vi "DrawGridOnMap.vi"(11 "Mission MapIn":picture) -> (3 "Mission MapOut":picture)   [LabVIEW 2014]
panel:
  out "decimal integer string":string
  out "Index":i32
  # "This Vi draws a grid on map with squares of N resolution"
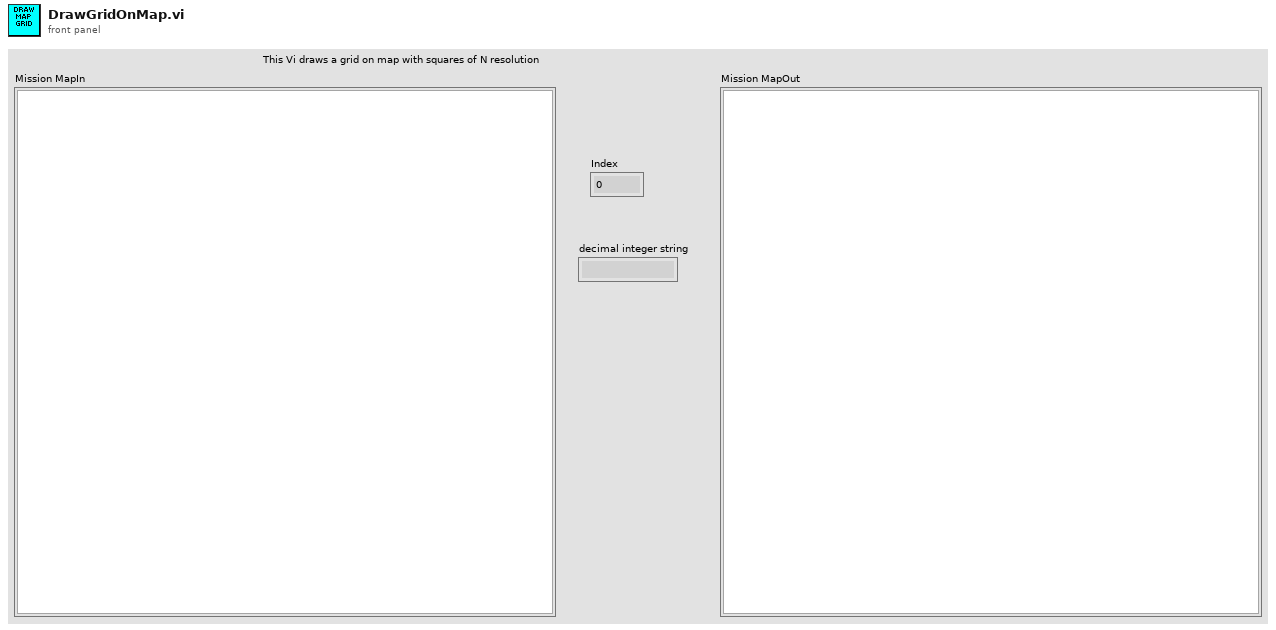
[diagram p1: front panel]
types:
  T1 = cluster{"Width":u16, "Style":enum32{"Solid", "Dash", "Dot", "DashDot", "DashDotDot"}}
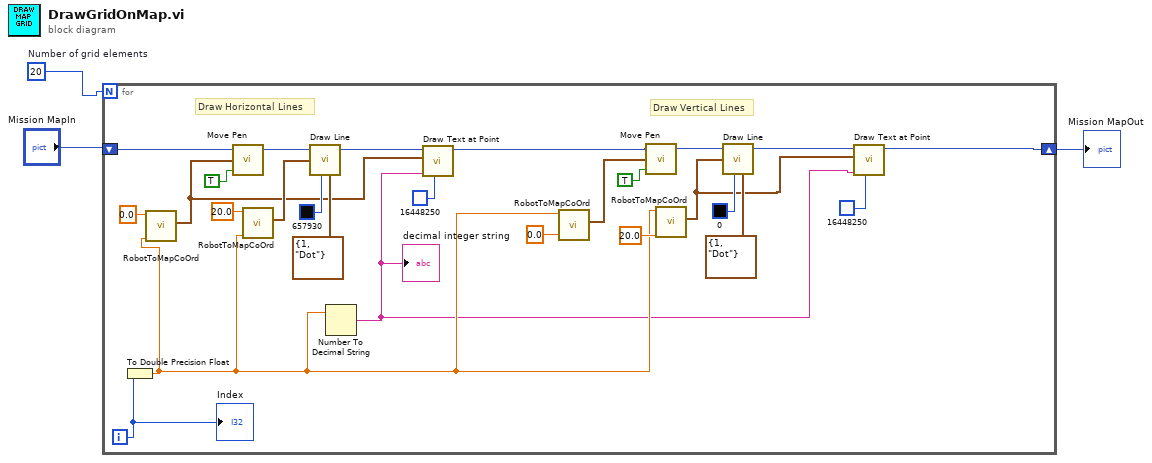
[diagram p0: block diagram]
diagram:
  w3 = 20  # Number of grid elements
  n1 = for {
    N: w3 -> [_]
    shift-right: [w8] -> w2
    shift-left: "Mission MapIn" -> [w22]
    i -> [w23]
    # "Draw Vertical Lines"
    # "Draw Horizontal Lines"
    n2 = To Double Precision Float(number=w23) -> (double precision float=w11:dbl)
    n3 = call "RobotToMapCoOrd.vi"("Robot Y"=w11, "Robot X"=0.0) -> ("RobotXandYonMap"=w10:cluster{"X":i32, "Y":i32})  [unwired: 9 in]
    n4 = call <vilib>:"Move Pen.vi"("absolute coordinates?(T)"=TRUE, "new position"=w10, "picture"=w22) -> ("new picture"=w29:picture)  [unwired: 2 in]
    n5 = call "RobotToMapCoOrd.vi"("Robot Y"=w11, "Robot X"=20.0) -> ("RobotXandYonMap"=w13:cluster{"X":i32, "Y":i32})  [unwired: 9 in]
    n6 = call <vilib>:"Draw Line.vi"("picture"=w29, "end point"=w13, "color(black)"=u32 657930, "pen"=T1 {"Width"=1, "Style"=enum."Dot"}) -> ("new picture"=w15:picture)  [unwired: 5 in]
    n7 = Number To Decimal String(number=w11) -> (decimal integer string=w7:string)  [unwired: 1 in]
    "decimal integer string" <- w7
    n8 = call <vilib>:"Draw Text at Point.vi"("text color(black)"=u32 16448250, "text"=w7, "origin"=w10, "picture"=w15) -> ("new picture"=w14:picture)  [unwired: 6 in, 1 out]
    n9 = call "RobotToMapCoOrd.vi"("Robot Y"=0.0 ("Robot X"), "Robot X"=w11) -> ("RobotXandYonMap"=w5:cluster{"X":i32, "Y":i32})  [unwired: 9 in]
    n10 = call <vilib>:"Move Pen.vi"("absolute coordinates?(T)"=TRUE, "new position"=w5, "picture"=w14) -> ("new picture"=w18:picture)  [unwired: 2 in]
    n11 = call "RobotToMapCoOrd.vi"("Robot Y"=20.0 ("Robot X"), "Robot X"=w11) -> ("RobotXandYonMap"=w4:cluster{"X":i32, "Y":i32})  [unwired: 9 in]
    n12 = call <vilib>:"Draw Line.vi"("picture"=w18, "end point"=w4, "color(black)"=u32 0, "pen"=T1 {"Width"=1, "Style"=enum."Dot"}) -> ("new picture"=w9:picture)  [unwired: 5 in]
    n13 = call <vilib>:"Draw Text at Point.vi"("text color(black)"=u32 16448250, "text"=w7, "origin"=w4, "picture"=w9) -> ("new picture"=w8:picture)  [unwired: 6 in, 1 out]
    "Index" <- w23
  }
  "Mission MapOut" <- w2
